vi "Wfm to Date and Time Arrays.vi"(6 "Save RPM Data":bool, 11 "Wfm In":waveform(dbl)) -> (0 "Time Strings":string[](array[string]), 1 "Date Strings":string[](array[string]))   [LabVIEW 2017]
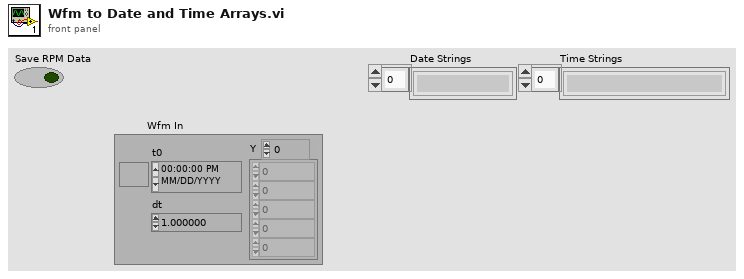
[diagram p1: front panel]
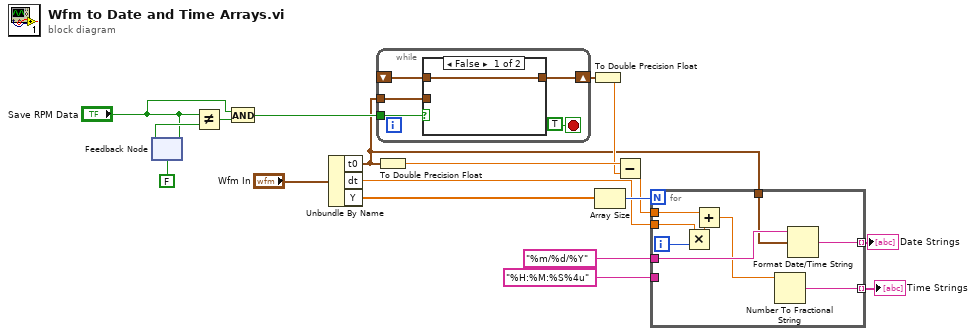
[diagram p0: block diagram]
diagram:
  n1 = feedback-in #1("Save RPM Data") -> ()
  n2 = feedback #1(FALSE) -> (w9:bool)
  n3 = Not Equal?(x="Save RPM Data", y=w9) -> (x != y?=w8:bool)
  n4 = And(x="Save RPM Data", y=w8) -> (x .and. y?=w6:bool)
  n5 = Unbundle By Name("Wfm In") -> ("t0"=w1:timestamp, "dt"=w15:dbl, "Y"=w17:dbl[])
  n6 = while {
    tunnel: w6 -> [w23]
    tunnel: w1 -> [w21]
    shift-right: [w20] -> w5
    shift-left: _ -> [w19]
    stop <- TRUE stop-if-true
    n7 = case shown="False" w23 {
      tunnel: w21 -> [_ w25]
      tunnel: [w24 w25] -> w20
      tunnel: w19 -> [w24 _]
      frame False {
      }
      frame True {
      }
    }
  }
  n8 = To Double Precision Float(number=w1) -> (double precision float=w4:dbl)
  n9 = To Double Precision Float(number=w5) -> (double precision float=w3:dbl)
  n10 = Array Size(array=w17) -> (size(s)=w16:i32)
  n11 = Subtract(x=w4, y=w3) -> (x-y=w2:dbl)
  n12 = for {
    N: w16 -> [_]
    tunnel: w2 -> [w31]
    tunnel: w15 -> [w33]
    tunnel: "%H:%M:%S%4u" -> [_]
    tunnel: "%m/%d/%Y" -> [w30]
    tunnel: [w29] -> w12 mode=indexing
    tunnel: [w26] -> w11 mode=indexing
    tunnel: w1 -> [w28]
    i -> [w34]
    n13 = Multiply(x=w33, y=w34) -> (x*y=w32:dbl)
    n14 = Add(x=w31, y=w32) -> (x+y=w27:dbl)
    n15 = Number To Fractional String(number=w27) -> (F-format string=w26:string)  [unwired: 3 in]
    n16 = Format Date/Time String(time format string (%c)=w30, seconds (now)=w28) -> (date/time string=w29:string)  [unwired: 1 in]
  }
  "Date Strings" <- w12
  "Time Strings" <- w11
